vi "Pour.vi"(8 "error in (no error)":errorcluster, 11 "Beer in":refnum<class "Beer.lvclass">) -> (0 "error out":errorcluster, 3 "Beer out":refnum<class "Beer.lvclass">)   [LabVIEW 2011, in "Beer.lvclass"]
uses:
  Beer.lvclass
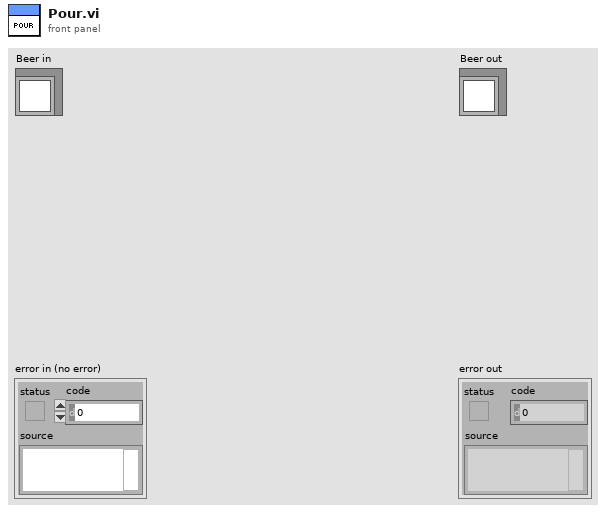
[diagram p1: front panel]
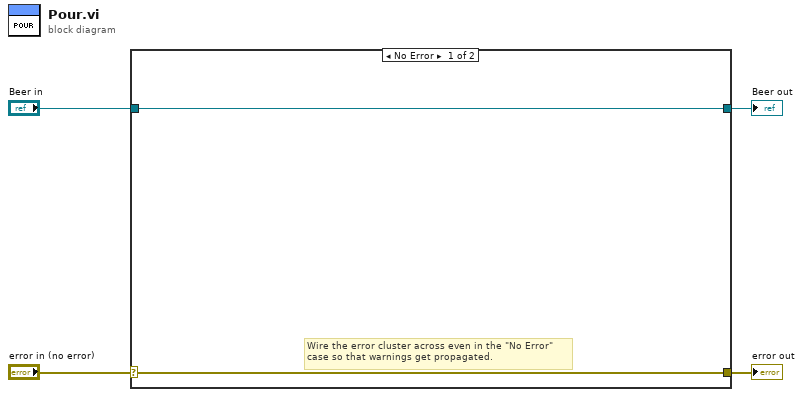
[diagram p0: block diagram]
diagram:
  n1 = case shown="No Error" "error in (no error)" {
    selector: "error in (no error)" -> [w5 w8]
    tunnel: [w5 w8] -> w3
    tunnel: [w6 w7] -> w1
    tunnel: "Beer in" -> [w6 w7]
    frame No Error {
      # "Wire the error cluster across even in the \"No Error\"\ncase so that warnings get propagated."
    }
    frame Error {
    }
  }
  "error out" <- w3
  "Beer out" <- w1
